vi "mVreader - Copy.vi"() -> (3 "Numeric":dbl)   [LabVIEW 2012]
panel:
  out "error out":errorcluster
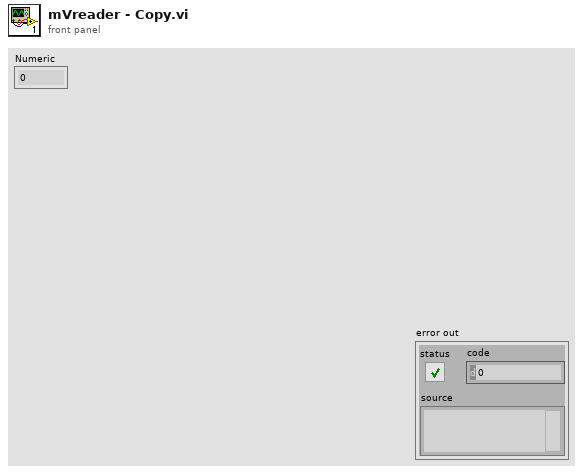
[diagram p1: front panel]
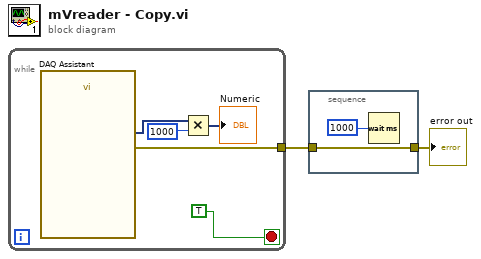
[diagram p0: block diagram]
diagram:
  n1 = while {
    tunnel: [w4] -> w1
    stop <- TRUE stop-if-true
    n2 = call "DAQ Assistant"() -> ("data"=w5:dynamicdata, "error out"=w4:errorcluster)  [unwired: 17 in, 1 out]
    n3 = Multiply(x=w5, y=1000) -> (x*y=→"Numeric":dynamicdata)
  }
  n4 = stacked-sequence {
    tunnel: w1 -> [w8]
    tunnel: [w8] -> w2
    frame #0 {
      n5 = Wait (ms)(milliseconds to wait=u32 1000) -> ()  [unwired: 1 out]
    }
  }
  "error out" <- w2
